vi "Vision Processing.vi"(4 "error in (no error)":errorcluster) -> ()   [LabVIEW 2011]
doc: "This VI runs in parallel to other tasks. It gets images from the camera, processes them for color or shape and use that information to affect robot behavior."
uses:
  Robot Global Data.vi
  <vilib>/gmath/NI_Gmath.lvlib
  <vilib>/gmath/interp.llb/Interpolate 2D (1d xi,yi).vi
panel:
  in  "Use Bin Detect":bool=TRUE
  in  "Distance":dbl[](array[numeric])=[0.0, 300.0]
  in  "Theta":dbl[](array[numeric])=[-90.0, 90.0]
  in  "Z":dbl[][](array[numeric])=[[0.0, 0.0], [0.0, 0.0]]
  out "Image":T1(plugin-control)
  out "deltay":dbl
  out "deltax":dbl
  out "distance":dbl
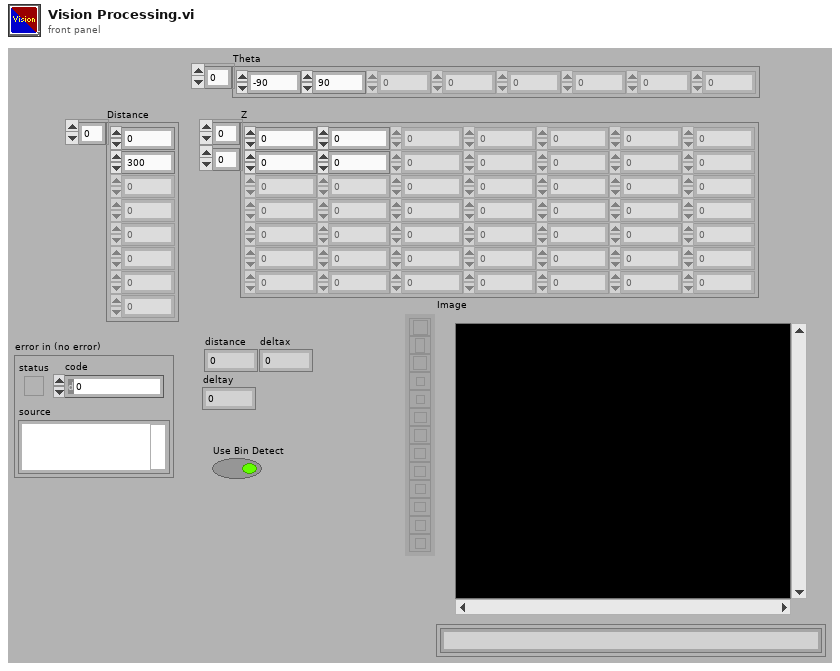
[diagram p1: front panel]
types:
  T1 = typedef "IMAQ Image.ctl" = refnum<image>
  T2 = typedef "Image Type" = u32
  T3 = typedef "WPI_CameraDevRef.ctl" = cluster{"Camera Address":string, "CameraStatus":errorcluster, "Acquire Image Notifier":refnum<notifier>}
  T4 = typedef "Semaphore RefNum" = refnum<k1>
  T5 = typedef "WPI_CameraImageSize.ctl" = enum16{"640x480", "320x240", "160x120"}
  T6 = cluster{"Aquire Target":bool, "Target Aquired":bool, "Attempts":dbl}
  T7 = typedef "CAN Data.ctl" = cluster{"Turret Position":dbl}
  T8 = typedef "Position Typedef.ctl" = cluster{"X":dbl, "Y":dbl, "Heading":dbl}
  T9 = typedef "Target Typedef.ctl" = cluster{"X":dbl, "Y":dbl, "Deltax":dbl, "Distance":dbl}
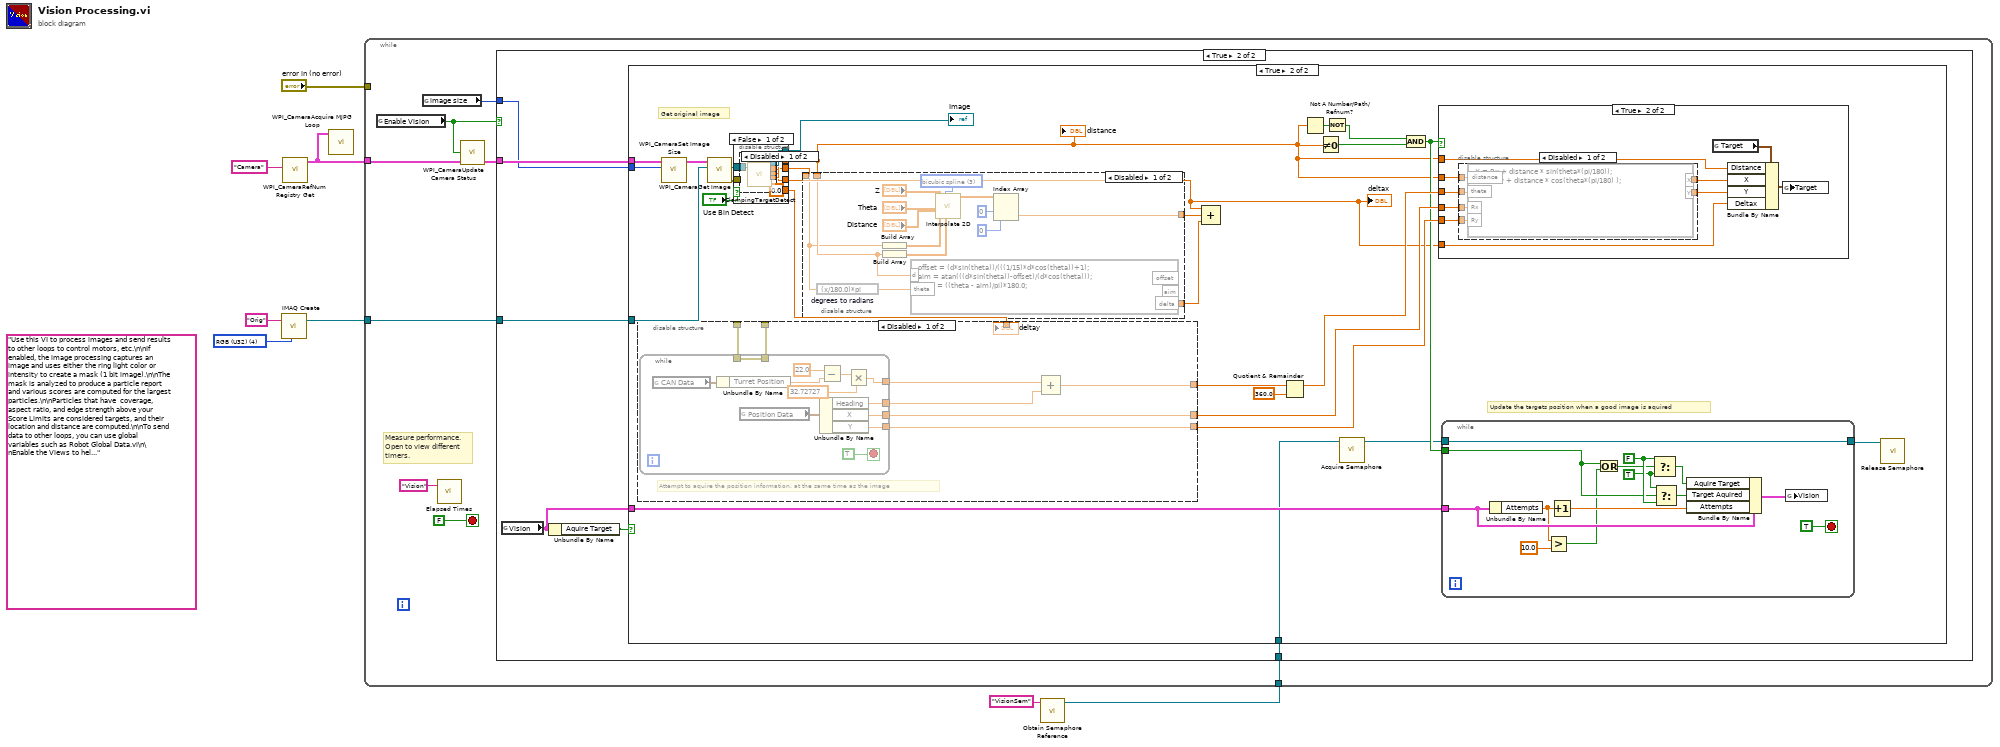
[diagram p0: block diagram]
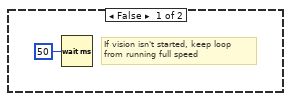
[diagram p2: hidden frame]
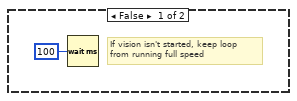
[diagram p3: hidden frame]
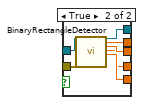
[diagram p5: hidden frame]
diagram:
  w6 = T2 4 items=["Grayscale (U8)", "Grayscale (I16)", "Grayscale (SGL)", "Complex (CSG)", "RGB (U32)", "HSL (U32)", "RGB (U64)", "Grayscale (U16)"] ("Image Type")
  (unwired) "Use this VI to process images and send results to other loops to control motors, etc.\n\nIf enabled, the image processing captures an image and uses either the ring light color or intensity to create a mask (1 bit image).\n\nThe mask is analyzed to produce a particle report and various scores are computed for the largest particles.\n\nParticles that have  coverage, aspect ratio, and edge strength above your Score Limits are considered targets, and their location and distance are computed.\n\nTo send data to other loops, you can use global variables such as Robot Global Data.vi\n\nEnable the Views to help debug color settings. Disable the View to speed up processing."
  n1 = call "IMAQ Create"("Image Name"="Orig", "Image Type"=w6) -> ("New Image"=w5:T1)  [unwired: 2 in, 2 out]
  n2 = call <vilib>:"WPI_CameraRefNum Registry Get.vi"("refnum name"="Camera") -> ("CameraDevRef"=w3:T3)  [unwired: 1 in, 9 out]
  n3 = call <vilib>:"WPI_CameraAcquire MJPG Loop.vi"("CameraDevRef"=w3) -> ()  [unwired: 11 in]
  n4 = call <vilib>:"Obtain Semaphore Reference.vi"("name (unnamed)"="VisionSem") -> ("semaphore"=w1:T4)  [unwired: 4 in, 2 out]
  n5 = while {
    tunnel: w5 -> [w15]
    tunnel: w3 -> [w14]
    tunnel: "error in (no error)" -> [_]
    tunnel: w1 -> [w9]
    stop <- FALSE stop-if-true
    # "Measure performance.\nOpen to view different\ntimers."
    n6 = global read "Robot Global Data.vi" "Enable Vision"() -> (w12:bool)
    n7 = global read "Robot Global Data.vi" "image size"() -> (w11:T5)
    n8 = call "Elapsed Times.vi"("Call Name"="Vision") -> ()  [unwired: 2 in, 1 out]
    n9 = call <vilib>:"WPI_CameraUpdate Camera Status.vi"("CameraDevRef In"=w14, "Enable Vision"=w12) -> ("CameraDevRef Out"=w13:T3)  [unwired: 3 in]
    n10 = case shown="True" w12 {
      tunnel: w15 -> [_ w23]
      tunnel: w13 -> [_ w22]
      tunnel: w11 -> [_ w21]
      tunnel: w9 -> [_ w18]
      frame False {
        # "If vision isn't started, keep loop\nfrom running full speed"
        n11 = Wait (ms)(milliseconds to wait=u32 50) -> ()  [unwired: 1 out]
      }
      frame True {
        n12 = global read "Robot Global Data.vi" "Vision"() -> (w19:T6)
        n13 = Unbundle By Name(w19) -> ("Aquire Target"=w20:bool)
        n14 = case shown="True" w20 {
          tunnel: w23 -> [_ w51]
          tunnel: w22 -> [_ w50]
          tunnel: w21 -> [_ w49]
          tunnel: w19 -> [_ w39]
          tunnel: w18 -> [_ w32]
          frame False {
            # "If vision isn't started, keep loop\nfrom running full speed"
            n15 = Wait (ms)(milliseconds to wait=u32 100) -> ()  [unwired: 1 out]
          }
          frame True {
            # "Update the targets position when a good image is aquired"
            # "Get original image"
            n16 = call <vilib>:"WPI_CameraSet Image Size.vi"("Image Size"=w49, "CameraDevRef"=w50) -> ("CameraDevRef Out"=w48:T3)  [unwired: 8 in, 1 out]
            n17 = call <vilib>:"WPI_CameraGet Image.vi"("Image"=w51, "CameraDevRef"=w48) -> ("error out"=w29:errorcluster, "Image Out"=w42:T1)  [unwired: 7 in, 1 out]
            n18 = case shown="False" "Use Bin Detect" {
              tunnel: w42 -> [w57 w69]
              tunnel: [0.0 ("deltay") w68] -> w41
              tunnel: [w56 w67] -> w37
              tunnel: [w55 w66] -> w31
              tunnel: [w54 w65] -> w30
              tunnel: w29 -> [_ w64]
              tunnel: [w53 w63] -> w26
              frame False {
                n19 = disable-structure shown="Disabled" {
                  disable-tunnel: w57 -> [w62 _]
                  disable-tunnel: [w61 _] -> w56
                  disable-tunnel: [w60 _] -> w55
                  disable-tunnel: [w59 _] -> w54
                  disable-tunnel: [w58 _] -> w53
                  frame Disabled {
                    n20 = call "ClampingTargetDetect.vi"("Image Src"=w62) -> ("Image Out"=w61:T1, "deltax"=w58:dbl, "theta"=w59:dbl, "distance"=w60:dbl)  [unwired: 14 in, 1 out]
                  }
                  frame Enabled {
                  }
                }
              }
              frame True {
                n21 = call "BinaryRectangleDetector.vi"("Image In"=w69, "error in"=w64) -> ("Image Out"=w67:T1, "distance"=w66:dbl, "theta"=w65:dbl, "deltax"=w63:dbl, "deltay"=w68:dbl)  [unwired: 20 in, 1 out]
              }
            }
            "distance" <- w31
            "deltax" <- w26
            "Image" <- w37
            n22 = disable-structure shown="Disabled" {
              disable-tunnel: [w91 _] -> w47
              disable-tunnel: _ -> [w90 _]
              disable-tunnel: [w87 _] -> w45
              disable-tunnel: [w86 _] -> w44
              disable-tunnel: [w85 _] -> _
              disable-tunnel: w41 -> [w84 _]
              frame Disabled {
                # "Attempt to aquire the position information, at the same time as the image"
                n23 = while {
                  tunnel: [w102] -> w88
                  tunnel: [w101] -> w85
                  tunnel: w90 -> [w101]
                  tunnel: [w93] -> w89
                  tunnel: [w98] -> w87
                  tunnel: [w97] -> w86
                  stop <- TRUE stop-if-true
                  n24 = global read "Robot Global Data.vi" "CAN Data"() -> (w99:T7)
                  n25 = Unbundle By Name(w99) -> ("Turret Position"=w92:dbl)
                  n26 = global read "Robot Global Data.vi" "Position Data"() -> (w103:T8)
                  n27 = Subtract(x=22.0, y=w92) -> (x-y=w96:dbl)
                  n28 = Unbundle By Name(w103) -> ("Heading"=w102:dbl, "X"=w98:dbl, "Y"=w97:dbl)
                  n29 = Multiply(x=w96, y=32.72727) -> (x*y=w93:dbl)
                }
                n30 = Compound Arithmetic op=ADD(w89, w88) -> (w91:dbl)  [unwired: 1 in]
                "deltay" <- w84
              }
              frame Enabled {
              }
            }
            n31 = disable-structure shown="Disabled" {
              disable-tunnel: w31 -> [w83 _]
              disable-tunnel: w30 -> [w81 _]
              disable-tunnel: [w80 _] -> w28
              disable-tunnel: [w79 _] -> w27
              frame Disabled {
                w75 = 3 items=["nearest", "bilinear", "bicubic", "bicubic spline"] ("method")
                n32 = expression code="(x/180.0)*pi" "degrees to radians"(w81) -> (w82:dbl)
                n33 = Build Array(w81) -> (w73:dbl[])
                n34 = Build Array(w83) -> (w74:dbl[])
                n35 = formula code="offset = (d*sin(theta))/(((1/15)*d*cos(theta))+1);\naim = atan(((d*sin(theta))-offset)/(d*cos(theta)));\ndelta = ((theta - aim)/pi)*180.0;"("d"=w83, "theta"=w82) -> ("delta"=w79:dbl)  [unwired: 2 out]
                n36 = call-poly <vilib>:"Interpolate 2D.vi"("yi"=w74, "method"=w75, "xi"=w73, "Y"="Distance", "X"="Theta", "Z"="Z") -> ("zi"=w72:dbl[][])  [unwired: 2 in, 3 out]
                n37 = Index Array(array=w72, index (row)=0, index (col)=0 ("disabled index (col)")) -> (element=w80:dbl)
              }
              frame Enabled {
              }
            }
            n38 = Compound Arithmetic op=ADD(w26, w28, w27) -> ()  [unwired: 1 out]
            n39 = Quotient & Remainder(x=w47, y=360.0) -> (x-y*floor(x/y)=w46:dbl)  [unwired: 1 out]
            n40 = Not A Number/Path/Refnum?(number/path/refnum=w31) -> (NaN/Path/Refnum?=w34:bool)
            n41 = Not Equal To 0?(x=w31) -> (x != 0?=w40:bool)
            n42 = Not(x=w34) -> (.not. x?=w33:bool)
            n43 = call <vilib>:"Acquire Semaphore.vi"("semaphore"=w32) -> ("semaphore out"=w36:T4)  [unwired: 4 in, 2 out]
            n44 = And(x=w33, y=w40) -> (x .and. y?=w38:bool)
            n45 = case shown="True" w38 {
              tunnel: w46 -> [_ w120]
              tunnel: w45 -> [_ w123]
              tunnel: w44 -> [_ w122]
              tunnel: w31 -> [_ w121]
              tunnel: w31 -> [_ w119]
              tunnel: w26 -> [_ w118]
              frame False {
              }
              frame True {
                n46 = disable-structure shown="Disabled" {
                  disable-tunnel: [w133 _] -> w126
                  disable-tunnel: [w132 _] -> w125
                  disable-tunnel: w123 -> [w131 _]
                  disable-tunnel: w122 -> [w130 _]
                  disable-tunnel: w121 -> [w129 _]
                  disable-tunnel: w120 -> [w128 _]
                  frame Disabled {
                    n47 = formula code="X = Rx + distance * sin(theta*(pi/180));\n   Y = Ry + distance * cos(theta*(pi/180) );"("Rx"=w131, "Ry"=w130, "distance"=w129, "theta"=w128) -> ("X"=w133:dbl, "Y"=w132:dbl)
                  }
                  frame Enabled {
                  }
                }
                n48 = global read "Robot Global Data.vi" "Target"() -> (w127:T9)
                n49 = Bundle By Name(cluster=w127, "Distance"=w119, "X"=w126, "Y"=w125, "Deltax"=w118) -> (w124:T9)
                n50 = global write "Robot Global Data.vi" "Target"(w124) -> ()
              }
            }
            n51 = while {
              tunnel: w39 -> [w117]
              tunnel: w38 -> [w105]
              tunnel: w36 -> [w109]
              tunnel: [w109] -> w35
              stop <- TRUE stop-if-true
              w112 = TRUE ("Target Aquired")
              w113 = FALSE ("Target Aquired")
              n52 = Unbundle By Name(w117) -> ("Attempts"=w108:dbl)
              n53 = Greater?(x=w108, y=10.0) -> (0:w104:bool)
              n54 = Increment(x=w108) -> (x+1=w115:dbl)
              n55 = Or(x=w105, y=w104) -> (x .or. y?=w106:bool)
              n56 = Select(t=w113, s=w106, f=w112) -> (s? t:f=w114:bool)
              n57 = Select(t=w112, s=w105, f=w113) -> (s? t:f=w111:bool)
              n58 = Bundle By Name(cluster=w117, "Aquire Target"=w114, "Target Aquired"=w111, "Attempts"=w115) -> (w116:T6)
              n59 = global write "Robot Global Data.vi" "Vision"(w116) -> ()
            }
            n60 = call <vilib>:"Release Semaphore.vi"("semaphore"=w35) -> ()  [unwired: 5 in, 2 out]
          }
        }
      }
    }
  }
